vi "timing.vi"(8 "error in (no error)":errorcluster, 10 "Timer Command":T1, 11 "Targe Time":i32) -> (0 "error out":errorcluster, 2 "Done?":bool, 3 "Elapsed Time":dbl)   [LabVIEW 2013]
uses:
  Controls/timer command.ctl
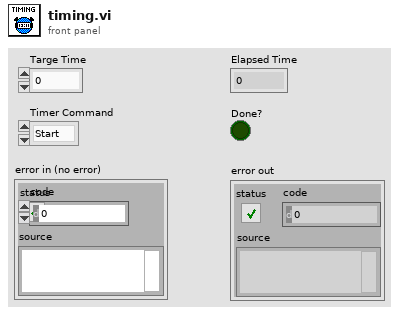
[diagram p1: front panel]
types:
  T1 = typedef "timer command.ctl" = enum16{"Start", "Check Time"}
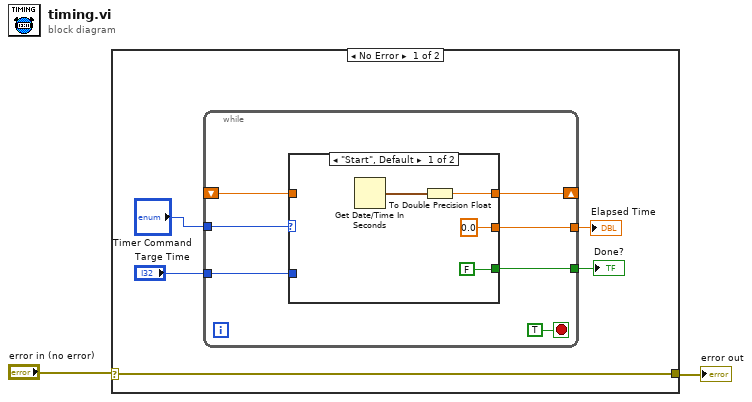
[diagram p0: block diagram]
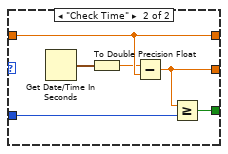
[diagram p2: hidden frame]
diagram:
  n1 = case shown="No Error" "error in (no error)" {
    selector: "error in (no error)" -> [w7 w25]
    tunnel: [w7 w25] -> w1
    frame No Error {
      n2 = while {
        tunnel: "Timer Command" -> [w14]
        shift-right: [w13] -> _
        shift-left: _ -> [w10]
        tunnel: [w12] -> w5
        tunnel: "Targe Time" -> [w9]
        tunnel: [w8] -> w3
        stop <- TRUE stop-if-true
        n3 = case shown="\"Start\", Default" w14 {
          tunnel: [w17 w23] -> w13
          tunnel: [0.0 w19] -> w12
          tunnel: w10 -> [_ w23]
          tunnel: w9 -> [_ w21]
          tunnel: [FALSE w20] -> w8
          frame "Start", Default {
            n4 = Get Date/Time In Seconds() -> (seconds since 1Jan1904=w18:timestamp)
            n5 = To Double Precision Float(number=w18) -> (double precision float=w17:dbl)
          }
          frame "Check Time" {
            n6 = Get Date/Time In Seconds() -> (seconds since 1Jan1904=w24:timestamp)
            n7 = To Double Precision Float(number=w24) -> (double precision float=w22:dbl)
            n8 = Subtract(x=w22, y=w23) -> (x-y=w19:dbl)
            n9 = Greater Or Equal?(x=w19, y=w21) -> (x >= y?=w20:bool)
          }
        }
      }
      "Elapsed Time" <- w5
      "Done?" <- w3
    }
    frame Error {
    }
  }
  "error out" <- w1
